vi "Write Serial Interface.vi"(8 "error in":errorcluster, 10 "Serial Interface":T1={"Baud Rate"=9600, "Data Bits "=8, "Parity"=enum."None", "Stop Bits"=0} {"Stop Bits" items=["1.0", "1.5", "2.0"]; "Baud Rate" items=["1200"=1200, "2400"=2400, "4800"=4800, "9600"=9600, "19200"=19200, "38400"=38400, "57600"=57600, "115200"=115200]}, 11 "VISA Interface in":refnum<class "VISA Interface.lvclass">) -> (0 "error out":errorcluster, 3 "VISA Interface out":refnum<class "VISA Interface.lvclass">)   [LabVIEW 2020, in "Plugin Instrument Driver.lvlib" / "VISA Interface.lvclass"]
doc: "Write Serial Interface"
uses:
  VISA Interface.lvclass
  builds/Libraries/Shared GUI Library.lvlibp/Shared GUI Library/Instrument Settings/Interface/Serial Interafce.ctl
  VISA Interface.lvclass/VISA Interface.ctl
  builds/Libraries/Shared GUI Library.lvlibp
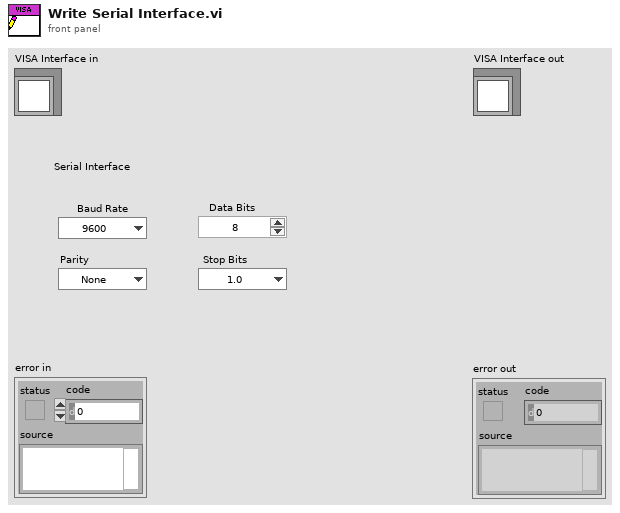
[diagram p1: front panel]
types:
  T1 = typedef "Shared GUI Library.lvlibp/Serial Interafce.ctl" = cluster{"Baud Rate":u32, "Data Bits ":u16, "Parity":enum16{"None", "Odd", "Even"}, "Stop Bits":u16}
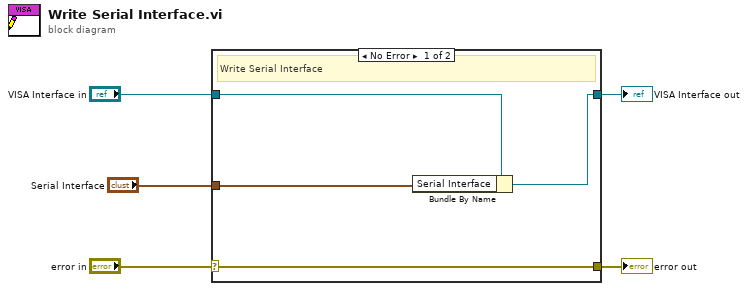
[diagram p0: block diagram]
diagram:
  n1 = case shown="No Error" "error in" {
    selector: "error in" -> [w9 w10]
    tunnel: [w9 w10] -> w4
    tunnel: [w7 w11] -> w2
    tunnel: "VISA Interface in" -> [w8 w11]
    tunnel: "Serial Interface" -> [w6 _]
    frame No Error {
      # "Write Serial Interface"
      n2 = Bundle By Name(cluster=w8, "Serial Interface"=w6) -> (w7:refnum<class "VISA Interface.lvclass">)
    }
    frame Error {
      # "Error"
    }
  }
  "error out" <- w4
  "VISA Interface out" <- w2
